vi "3458A Initialize Virtual Channels.vi"(8 "error in":errorcluster, 10 "reset instruments (False)":bool, 11 "digitizer in":T1={"channels"=[], "sync unit"={"VISA"="", "type"=enum."Picotest U6200A"}, "awg unit"={"type"=enum."Agilent 331xxA to 332xxA", "VISA"="", "enable 10MHz ref"=FALSE}, "sync mode"=enum."MASTER-SLAVE, MASTER clocked by TIMER", "streaming mode"=FALSE, "idn mode"=enum."Auto", "sampling mode"=enum."DCV", "Ts [s]"=0.0, "sample memory [B]"=0, "proc setup"={"channel id"=0, "packet size [smpl]"=0, "current timeout [s]"=0.0, "blk2blk timeout [s]"=0.0, "event time"=timestamp(0 s since 1904-01-01), "stop notifier"=refnum, "data queues"=[], "proc refs"=[], "bus semaphore"=refnum}, "sample size [B]"=0, "sample count"=0, "aux data"={"channel id"=0, "valid?"=[], "gain [V]"=[], "timestamp [s]"=[], "Ts [s]"=0.0, "abs timestamp"=timestamp(0 s since 1904-01-01), "t [deg C]"=[], "multiplex timestamp [s]"=-1.0, "only multiplex?"=FALSE, "multiplex smpl offset"=0}, "ranges [V]"=[], "aperture [s]"=0.0, "LEVEL trigger"={"edge"=enum."POS", "level [V]"=0.0, "coupling"=enum."DC"}, "trigger mode"=enum."AUTO", "measure temp.?"=FALSE, "disp mesages"=[], "shared bus?"=FALSE, "disable display?"=FALSE, "aper mode"=enum."Manual", "aper rules"=[], "multiplex"={"cycles"=0, "delay [s]"=0.0, "enabled"=FALSE, "overhead [s]"=1.0, "tot smpls"=0, "sub-rec"=0, "overhead [%]"=0.0}, "F8588 lpf"=enum."Off"} {"channels"."Range [Vpk]" min=0.0}) -> (0 "error out":errorcluster, 1 "awg idn string":string, 2 "dmm(s) idn strings":string[](array[string]), 3 "digitizer out":T1={"channels"=[], "sync unit"={"VISA"="", "type"=enum."Picotest U6200A"}, "awg unit"={"type"=enum."Agilent 331xxA to 332xxA", "VISA"="", "enable 10MHz ref"=FALSE}, "sync mode"=enum."MASTER-SLAVE, MASTER clocked by TIMER", "streaming mode"=FALSE, "idn mode"=enum."Auto", "sampling mode"=enum."DCV", "Ts [s]"=0.0, "sample memory [B]"=0, "proc setup"={"channel id"=0, "packet size [smpl]"=0, "current timeout [s]"=0.0, "blk2blk timeout [s]"=0.0, "event time"=timestamp(0 s since 1904-01-01), "stop notifier"=refnum, "data queues"=[], "proc refs"=[], "bus semaphore"=refnum}, "sample size [B]"=0, "sample count"=0, "aux data"={"channel id"=0, "valid?"=[], "gain [V]"=[], "timestamp [s]"=[], "Ts [s]"=0.0, "abs timestamp"=timestamp(0 s since 1904-01-01), "t [deg C]"=[], "multiplex timestamp [s]"=-1.0, "only multiplex?"=FALSE, "multiplex smpl offset"=0}, "ranges [V]"=[], "aperture [s]"=0.0, "LEVEL trigger"={"edge"=enum."POS", "level [V]"=0.0, "coupling"=enum."DC"}, "trigger mode"=enum."AUTO", "measure temp.?"=FALSE, "disp mesages"=[], "shared bus?"=FALSE, "disable display?"=FALSE, "aper mode"=enum."Manual", "aper rules"=[], "multiplex"={"cycles"=0, "delay [s]"=0.0, "enabled"=FALSE, "overhead [s]"=1.0, "tot smpls"=0, "sub-rec"=0, "overhead [%]"=0.0}, "F8588 lpf"=enum."Off"} {"channels"."Range [Vpk]" min=0.0}, 4 "sync unit idn string":string)   [LabVIEW 2013, in "3458A Virtual Digitizer.lvlib"]
doc: "Call this to open all intruments related to the digitizing DMMs system.\n1) Opens all 3458A channels.\n2) If needed for selected mode, opens counter for measurement of two channels time shift (used for 3458A with synchronized clocks).\n3) If needed for selected mode, opens AWG."
uses:
  3458A Virtual Digitizer.lvlib
  3458A Digitizer Session.ctl
  3458A Virtual Channel Config.ctl
  Counter/Counter Session.ctl
  Counter/Counter Type.ctl
  AWG/AWG Session.ctl
  AWG/AWG Type.ctl
  3458A Sync Mode.ctl
  3458A Idn Mode.ctl
  3458A Digitizing Low Levels/Configure/Sampling Mode.ctl
  3458A Digitizing Process Options.ctl
  3458A Data Packet.ctl
  3458A Aux Record Data.ctl
  3458A Digitizing Low Levels/Configure/Level Setup.ctl
  3458A Digitizing Low Levels/Configure/First Sample Trigger.ctl
  3458A Aperture Selection Mode.ctl
  3458A Multiplexing Config.ctl
  Fluke 8588A/F8588A Low Pass Filter.ctl
  3458A Digitizing Low Levels/3458A Digitizing Low Levels.lvlib
  AWG/AWG.lvlib
  Counter/Counter.lvlib
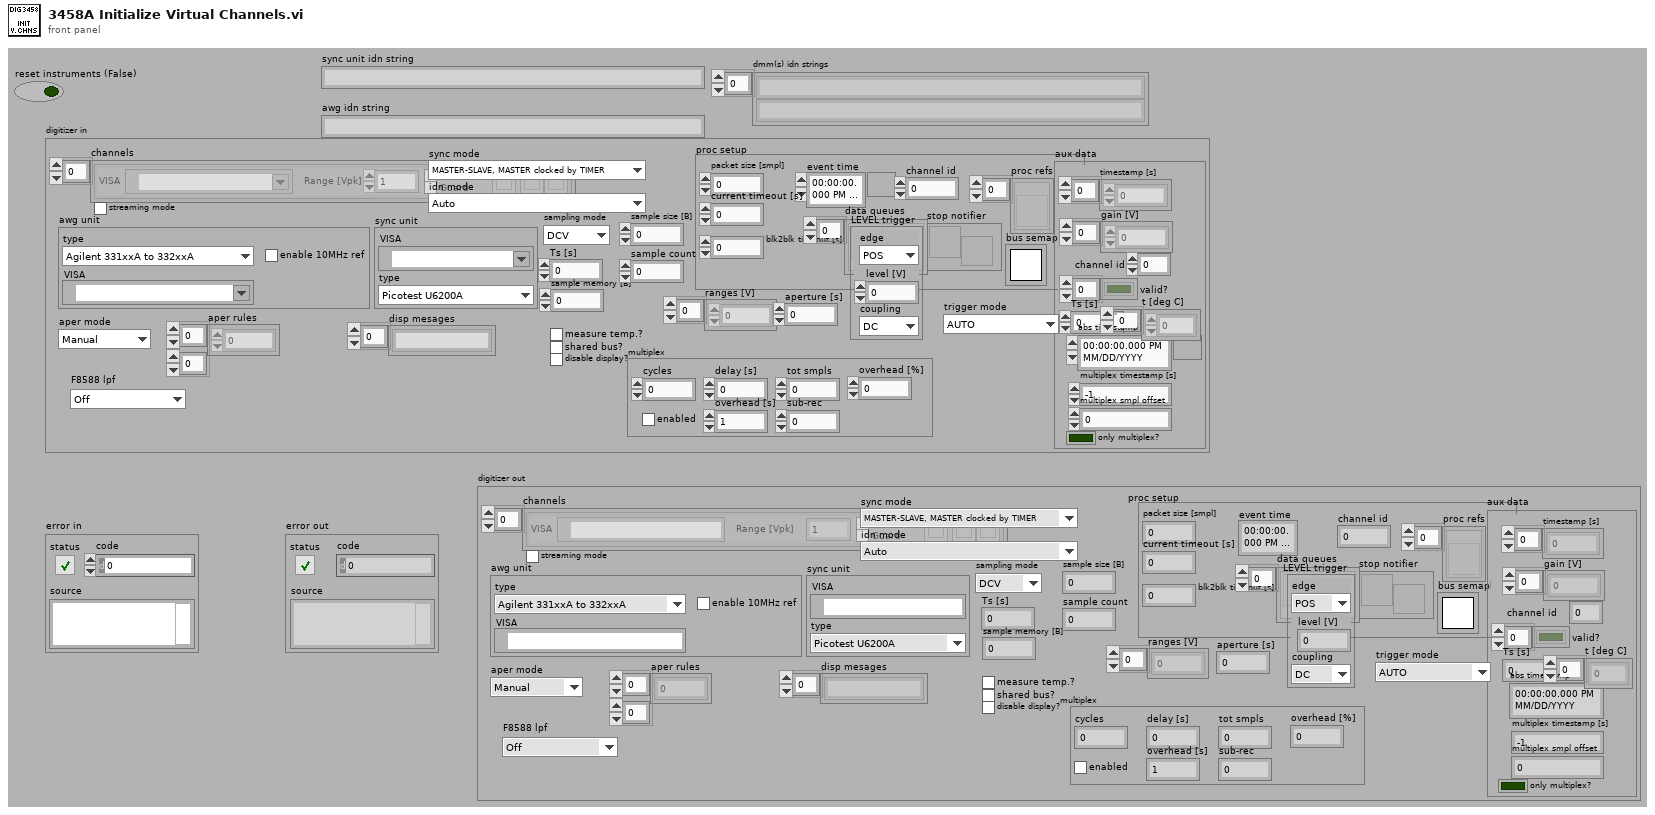
[diagram p1: front panel]
types:
  T1 = typedef "3458A Virtual Digitizer.lvlib/3458A Digitizer Session.ctl" = cluster{"channels":T2[], "sync unit":T3, "awg unit":T5, "sync mode":T7, "streaming mode":bool, "idn mode":T8, "sampling mode":T9, "Ts [s]":dbl, "sample memory [B]":i32, "proc setup":T10, "sample size [B]":i32, "sample count":i32, "aux data":T12, "ranges [V]":dbl[], "aperture [s]":dbl, "LEVEL trigger":T13, "trigger mode":T14, "measure temp.?":bool, "disp mesages":string[], "shared bus?":bool, "disable display?":bool, "aper mode":T15, "aper rules":dbl[][], "multiplex":T16, "F8588 lpf":T17}
  T2 = typedef "3458A Virtual Digitizer.lvlib/3458A Virtual Channel Config.ctl" = cluster{"VISA":refnum<visa-resource-name>, "Range [Vpk]":dbl, "btn clr":bool, "btn up":bool, "btn down":bool, "F8588":bool, "F8588 guard":bool}
  T3 = typedef "Counter.lvlib/Counter Session.ctl" = cluster{"VISA":refnum<visa-resource-name>, "type":T4}
  T4 = typedef "Counter.lvlib/Counter Type.ctl" = enum16{"Picotest U6200A", "dummy"}
  T5 = typedef "AWG.lvlib/AWG Session.ctl" = cluster{"type":T6, "VISA":refnum<visa-resource-name>, "enable 10MHz ref":bool}
  T6 = typedef "AWG.lvlib/AWG Type.ctl" = enum16{"Agilent 331xxA to 332xxA", "Agilent 335xxA to 336xxA", "Tektronix AFG3101C", "dummy"}
  T7 = typedef "3458A Virtual Digitizer.lvlib/3458A Sync Mode.ctl" = enum16{"MASTER-SLAVE, MASTER clocked by TIMER", "MASTER-SLAVE, MASTER clocked by AWG", "ALL clocked by AWG", "MASTER-SLAVE, ALL clocked by TIMER", "ALL clocked by AWG with DFLL"}
  T8 = typedef "3458A Virtual Digitizer.lvlib/3458A Idn Mode.ctl" = enum16{"Auto", "Sequential (chn A, chn B, ...)", "From calibration string"}
  T9 = typedef "3458A Virtual Digitizer.lvlib/3458A Digitizing Low Levels.lvlib/Sampling Mode.ctl" = enum16{"DCV", "DSDC", "DSAC"}
  T10 = typedef "3458A Virtual Digitizer.lvlib/3458A Digitizing Process Options.ctl" = cluster{"channel id":i32, "packet size [smpl]":i32, "current timeout [s]":dbl, "blk2blk timeout [s]":dbl, "event time":timestamp, "stop notifier":refnum<notifier>, "data queues":refnum<queue>[], "proc refs":refnum<vi>[], "bus semaphore":T11}
  T11 = typedef "Semaphore RefNum" = refnum<k1>
  T12 = typedef "3458A Virtual Digitizer.lvlib/3458A Aux Record Data.ctl" = cluster{"channel id":i32, "valid?":bool[], "gain [V]":dbl[], "timestamp [s]":dbl[], "Ts [s]":dbl, "abs timestamp":timestamp, "t [deg C]":dbl[], "multiplex timestamp [s]":dbl, "only multiplex?":bool, "multiplex smpl offset":i64}
  T13 = typedef "3458A Virtual Digitizer.lvlib/3458A Digitizing Low Levels.lvlib/Level Setup.ctl" = cluster{"edge":enum16{"POS", "NEG"}, "level [V]":dbl, "coupling":enum16{"DC", "AC"}}
  T14 = typedef "3458A Virtual Digitizer.lvlib/3458A Digitizing Low Levels.lvlib/First Sample Trigger.ctl" = enum16{"AUTO", "EXT", "SYN", "SGL", "HOLD", "LEVEL"}
  T15 = typedef "3458A Virtual Digitizer.lvlib/3458A Aperture Selection Mode.ctl" = enum16{"Manual", "Maximum", "Table"}
  T16 = typedef "3458A Multiplexing Config.ctl" = cluster{"cycles":i32, "delay [s]":dbl, "enabled":bool, "overhead [s]":dbl, "tot smpls":i64, "sub-rec":i32, "overhead [%]":dbl}
  T17 = typedef "F8588A Low Pass Filter.ctl" = enum16{"Off", "100 kHz", "3 MHz"}
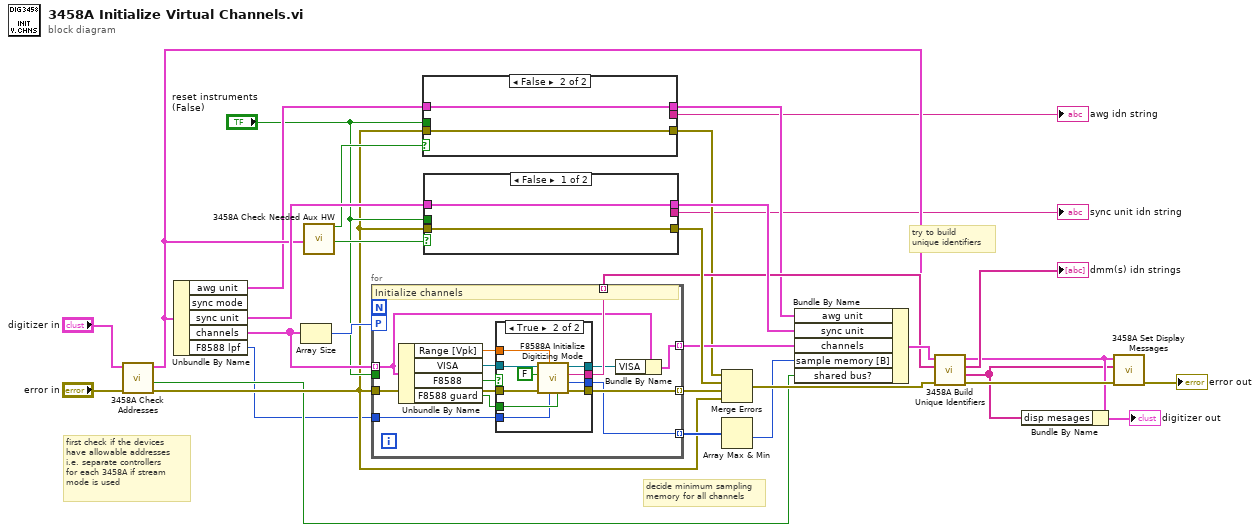
[diagram p0: block diagram]
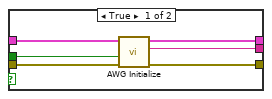
[diagram p2: hidden frame]
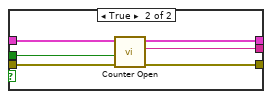
[diagram p3: hidden frame]
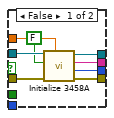
[diagram p4: hidden frame]
diagram:
  # "decide minimum sampling\nmemory for all channels"
  # "try to build\nunique identifiers"
  # "first check if the devices\nhave allowable addresses\ni.e. separate controllers\nfor each 3458A if stream\nmode is used"
  n1 = call "3458A Check Addresses.vi"("error in"="error in", "digitizer session in"="digitizer in") -> ("error out"=w3:errorcluster, "some dmms shares the same controller?"=w2:bool, "digitizer session out"=w18:T1)  [unwired: 6 in, 1 out]
  n2 = Unbundle By Name(w18) -> ("awg unit"=w17:T5, "sync unit"=w29:T3, "channels"=w32:T2[], "F8588 lpf"=w1:T17)  [unwired: 1 out]
  n3 = Array Size(array=w32) -> (size(s)=w31:i32)
  n4 = call "3458A Check Needed Aux HW.vi"("digitizer session"=w18) -> ("uses AWG clocking?"=w15:bool, "uses counter?"=w16:bool)  [unwired: 13 in, 4 out]
  n5 = for {
    tunnel: w3 -> [w44]
    tunnel: w32 -> [w39] mode=indexing
    workers-P: w31 -> [_]
    tunnel: [w43] -> w30 mode=indexing
    tunnel: [w38] -> w26 mode=indexing
    tunnel: [w42] -> w21 mode=indexing
    tunnel: "reset instruments (False)" -> [_]
    tunnel: [w37] -> w20 mode=indexing
    tunnel: w1 -> [w33]
    # "Initialize channels"
    n6 = Unbundle By Name(w39) -> ("Range [Vpk]"=w36:dbl, "VISA"=w41:refnum<visa-resource-name>, "F8588"=w35:bool, "F8588 guard"=w34:bool)
    n7 = case shown="True" w35 {
      tunnel: w44 -> [w52 w62]
      tunnel: [w51 w61] -> w43
      tunnel: [w50 w56] -> w42
      tunnel: w41 -> [w49 w60]
      tunnel: [w48 w57] -> w40
      tunnel: [w47 w55] -> w37
      tunnel: w36 -> [w45 w58]
      tunnel: w34 -> [_ w54]
      tunnel: w33 -> [_ w53]
      frame False {
        n8 = call "Initialize 3458A.vi"("range [V] (10V)"=w45, "error in (no error)"=w52, "Reset (True)"=FALSE, "VISA DMM"=w49) -> ("error out"=w51:errorcluster, "sample memory [B]"=w47:i32, "idn string"=w50:string, "VISA resource name out"=w48:refnum<visa-resource-name>)  [unwired: 4 in]
      }
      frame True {
        n9 = call "F8588A Initialize Digitizing Mode.vi"("Ext Guard (false)"=w54, "Low Pass Filter (off)"=w53, "range [V] (10V)"=w58, "error in (no error)"=w62, "Reset (True)"=FALSE, "VISA DMM"=w60) -> ("error out"=w61:errorcluster, "sample memory [B]"=w55:i32, "idn string"=w56:string, "VISA resource name out"=w57:refnum<visa-resource-name>)  [unwired: 2 in]
      }
    }
    n10 = Bundle By Name(cluster=w39, "VISA"=w40) -> (w38:T2)
  }
  n11 = case shown="False" w15 {
    tunnel: w3 -> [w68 w70]
    tunnel: [w65 w70] -> w14
    tunnel: w17 -> [w67 w69]
    tunnel: [w66 w69] -> w13
    tunnel: [w64 _] -> w12
    tunnel: "reset instruments (False)" -> [w63 _]
    frame True {
      # "Initialize AWG"
      n12 = call "AWG Initialize.vi"("error in (no error)"=w68, "Reset (True)"=w63, "awg session in"=w67) -> ("error out"=w65:errorcluster, "idn string"=w64:string, "awg session out"=w66:T5)  [unwired: 6 in]
    }
    frame False {
    }
  }
  "awg idn string" <- w12
  n13 = case shown="False" w16 {
    tunnel: w3 -> [w71 w78]
    tunnel: w29 -> [w72 w77]
    tunnel: [w71 w75] -> w28
    tunnel: [w72 w73] -> w27
    tunnel: "reset instruments (False)" -> [_ w76]
    tunnel: [_ w74] -> w10
    frame False {
      # "Initialize AWG"
    }
    frame True {
      # "Initialize counter"
      n14 = call "Counter Open.vi"("error in"=w78, "Reset (True)"=w76, "couner session in"=w77) -> ("error out"=w75:errorcluster, "idn string"=w74:string, "counter session out"=w73:T3)  [unwired: 6 in]
    }
  }
  "sync unit idn string" <- w10
  n15 = Merge Errors(w14, w28, w30, w3) -> (w23:errorcluster)
  n16 = Array Max & Min(array=w20) -> (min value=w19:i32)  [unwired: 3 out]
  n17 = Bundle By Name(cluster=w18, "awg unit"=w13, "sync unit"=w27, "channels"=w26, "sample memory [B]"=w19, "shared bus?"=w2) -> (w22:T1)
  n18 = call "3458A Build Unique Identifiers.vi"("error in"=w23, "dmm(s) idn strings in"=w21, "digitizer session in"=w22) -> ("error out"=w9:errorcluster, "display strings"=w5:string[], "identifier strings"=→"dmm(s) idn strings":string[], "digitizer session out"=w6:T1)  [unwired: 5 in]
  n19 = Bundle By Name(cluster=w6, "disp mesages"=w5) -> (→"digitizer out":T1)
  n20 = call "3458A Set Display Messages.vi"("error in (no error)"=w9, "display strings"=w5, "digitizer session in"=w6) -> ("error out"=→"error out":errorcluster)  [unwired: 7 in, 1 out]
